vi "global_variables_AWG.vi"() -> ()   [LabVIEW 2014]
panel:
  out "y-magnet 2":dbl
  out "z-magnet 2":dbl=20.0
  in  "Last magnet position":path=path "C:/Users/C4.1a/Desktop/Labview VIs/ODMRmagnetConex/ConexCC/last_magnet_position.txt"
  out "laser voltage":dbl
  out "z-magnet":dbl=6.704
  out "y-magnet":dbl=8.468
  out "x-magnet":dbl=19.643
  out "z-position":dbl=4.365591397849463
  out "y-position":dbl=-0.4473684210526316
  out "x-position":dbl=-0.014970059880239564
  in  "Last Scan":path=path "C:/Users/C4.1a/Desktop/Tobias/data/raw data/2011-12-01_11-41-50_248.txt"
  in  "pulse program index":u32
  in  "start trigger cycles":u32=50
  in  "start trigger marker channel":u32=3
  in  "signal marker channel":u32=1
  in  "#phase cycles":u32=1
  in  "constants":dbl[](array[numeric])=[0.0001] format="%#_6p"
  in  "AWG carrier frequency":ext=100000000.0 format="%#_6p"
  in  "AWG sampling frequency":ext=500000000.0 format="%#_6p"
  in  "awg line":T1 {"phase" format="%.3f"; "amplitude" format="%.3f"; "time" format="%#_6p"}
  in  "variables":dbl[][](array[numeric])=[[1e-07], [3e-07], [5e-07], [1e-06], [3e-06], [5e-06], [1e-05], [3e-05], [5e-05], [0.0001], [0.0003], [0.0005], [0.001], [0.003]]
  in  "loop index":u32=59
  # "default: 1"
  # "default: 0"
  # "default: 500MHz"
  # "default: 100MHz"
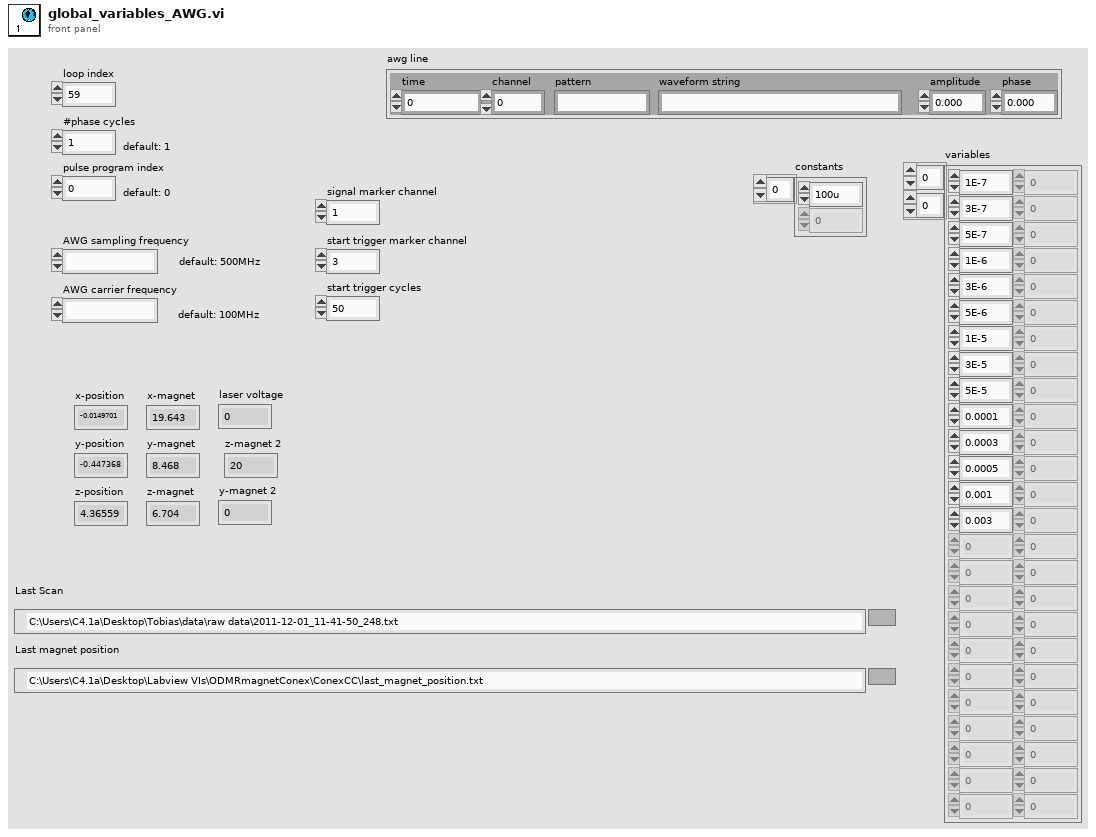
[diagram p1: front panel]
types:
  T1 = cluster{"time":ext, "channel":i32, "pattern":string, "waveform string":string, "amplitude":ext, "phase":ext}
diagram:
